vi "Cal Rate.vi"(8 "error in (no error)":errorcluster, 11 "Automation in":refnum<class "NMR Data.lvclass">) -> (0 "error out":errorcluster, 2 "mean Rate":dbl format="%.9f", 3 "Automation out":refnum<class "NMR Data.lvclass">)   [LabVIEW 2019, in "NMR Data.lvclass"]
uses:
  NMR Data.lvclass
  NMR Data.lvclass/NMR Data.ctl
  <vilib>/Analysis/baseanly.llb/Mean (DBL).vi
  <vilib>/Analysis/NI_AALBase.lvlib
panel:
  out "Slopes":dbl[](array[numeric])
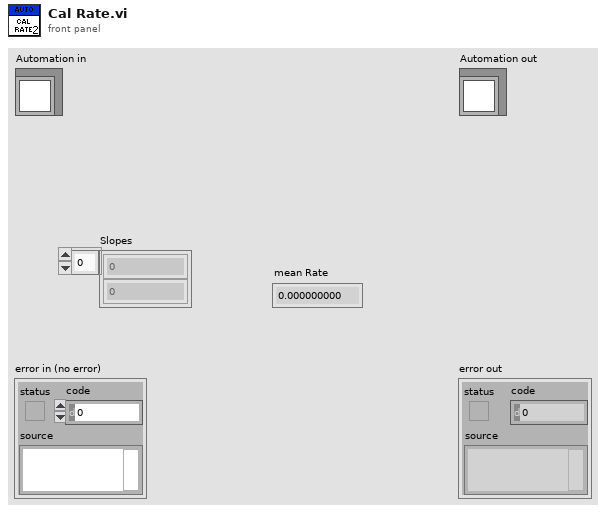
[diagram p1: front panel]
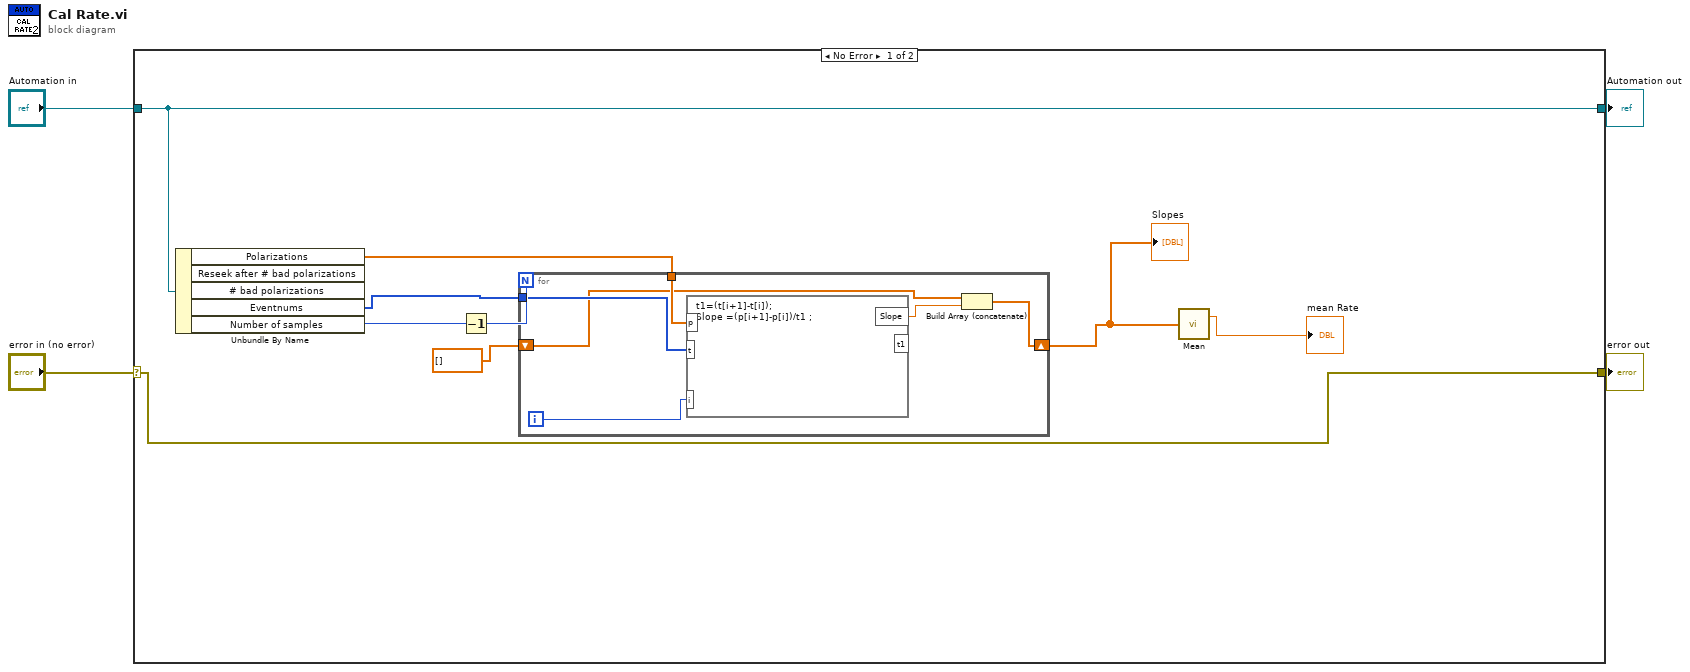
[diagram p0: block diagram]
diagram:
  n1 = case shown="No Error" "error in (no error)" {
    selector: "error in (no error)" -> [w5 w21]
    tunnel: [w10 w20] -> w2
    tunnel: "Automation in" -> [w10 w20]
    tunnel: [w5 w21] -> w1
    frame No Error {
      n2 = Unbundle By Name(w10) -> ("Polarizations"=w6:dbl[], "Eventnums"=w8:i64[], "Number of samples"=w9:i32)  [unwired: 2 out]
      n3 = Decrement(x=w9) -> (x-1=w13:i32)
      n4 = for {
        N: w13 -> [_]
        tunnel: w6 -> [w19]
        tunnel: w8 -> [w18]
        shift-right: [w14] -> w12
        shift-left: dbl[] [] ("appended array") -> [w15]
        i -> [w17]
        n5 = formula code="t1=(t[i+1]-t[i]);\nSlope =(p[i+1]-p[i])/t1 ;"("p"=w19, "t"=w18, "i"=w17) -> ("Slope"=w16:dbl)  [unwired: 1 out]
        n6 = Build Array (concatenate)(w15, w16) -> (w14:dbl[])
      }
      "Slopes" <- w12
      n7 = call-poly <vilib>:"Mean.vi"("X"=w12) -> ("mean"=→"mean Rate":dbl)  [unwired: 1 out]
    }
    frame Error {
    }
  }
  "error out" <- w1
  "Automation out" <- w2
